vi "CREATE USER.vi"() -> ()   [LabVIEW 2021]
panel:
  in  "Cancel Button":bool
  in  "OK Button":bool
  in  "CONFIRM PASSWORD":string
  in  "PASSWORD":string
  in  "USER NAME":string
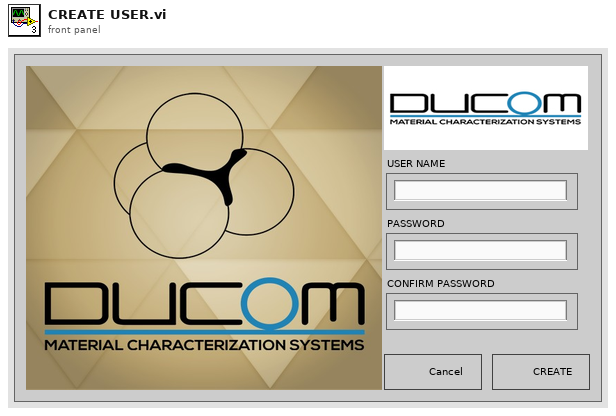
[diagram p1: front panel]
types:
  T1 = enum8{"Enabled", "Disabled", "Disabled and Grayed Out"}
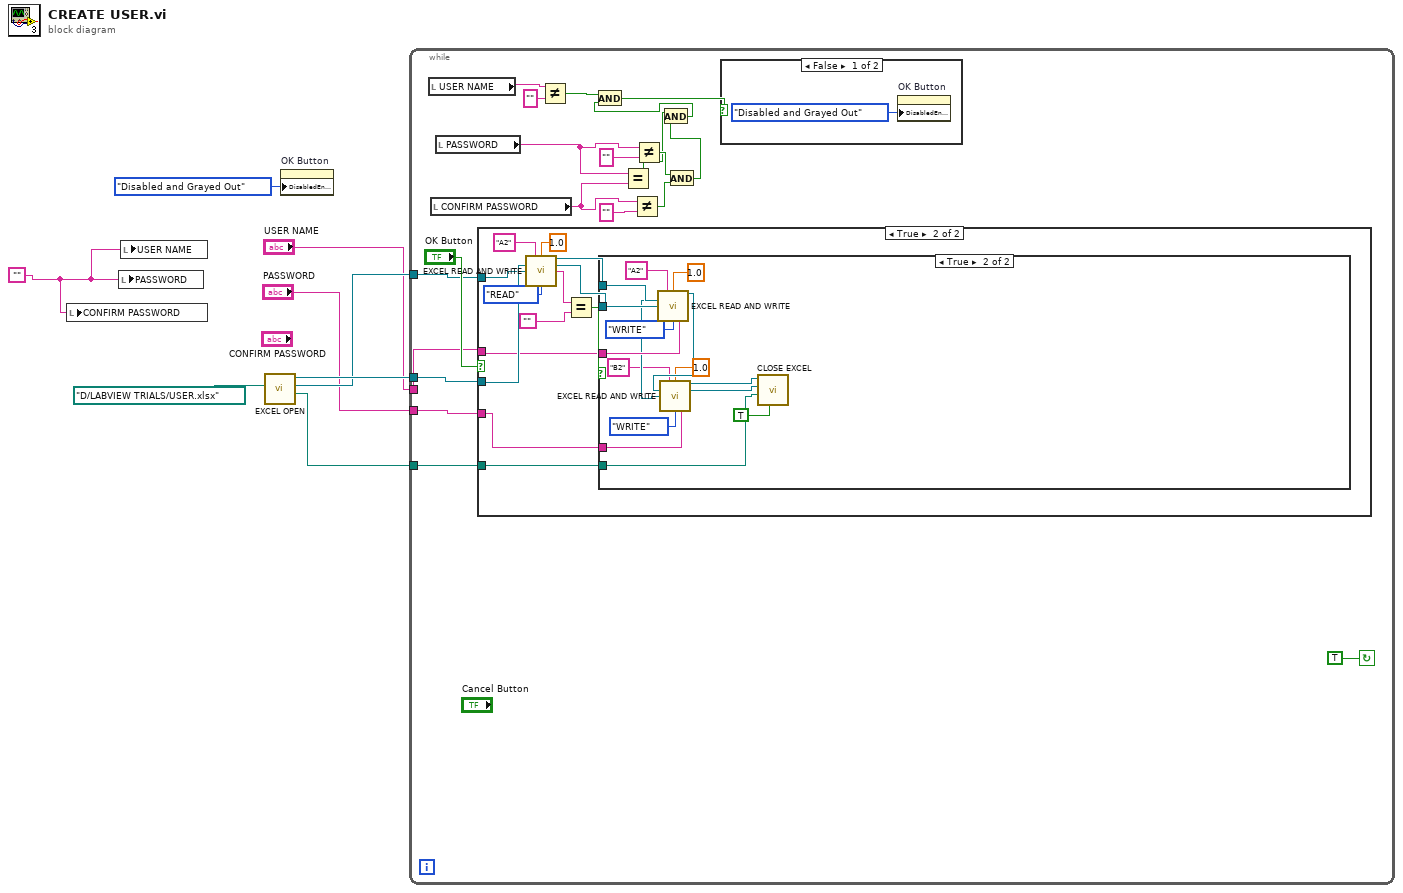
[diagram p0: block diagram]
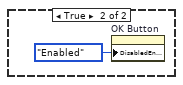
[diagram p4: hidden frame]
diagram:
  w7 = ""
  n1 = local write "CONFIRM PASSWORD"(w7) -> ()
  n2 = local write "PASSWORD"(w7) -> ()
  n3 = local write "USER NAME"(w7) -> ()
  n4 = call "EXCEL OPEN.vi"("PATH IN"=path "D:/LABVIEW TRIALS/USER.xlsx") -> ("PATH OUT"=w1:path, "WORKBOOK OUT"=w4:refnum<k7>, "Excel Application ref  out"=w5:refnum<k7>)  [unwired: 6 in, 2 out]
  n5 = property on="OK Button" class="Bool"("DisabledEnum"=T1."Disabled and Grayed Out" ("Disabled")) -> ()  [unwired: 2 in, 2 out]
  n6 = while {
    tunnel: w5 -> [w13]
    tunnel: w4 -> [w12]
    tunnel: "USER NAME" -> [w11]
    tunnel: "PASSWORD" -> [w10]
    tunnel: w1 -> [w9]
    stop <- TRUE continue-if-true
    n7 = local read "USER NAME"() -> (w17:string)
    n8 = local read "CONFIRM PASSWORD"() -> (w15:string)
    n9 = local read "PASSWORD"() -> (w16:string)
    n10 = case shown="True" "OK Button" {
      tunnel: w13 -> [_ w41]
      tunnel: w12 -> [_ w40]
      tunnel: w11 -> [_ w31]
      tunnel: w10 -> [_ w30]
      tunnel: w9 -> [_ w29]
      frame False {
      }
      frame True {
        n11 = call "EXCEL READ AND WRITE.vi"("CELL"="A2", "SHEET INDEX"=1.0, "Excel.Application REF in"=w41, "Excel._Workbook"=w40, "OPERATION"=enum16{"READ", "WRITE"}."READ") -> ("Excel Application ref out"=w33:refnum<k7>, "WORKBOOK REF OUT"=w32:refnum<k7>, "READING FROM EXCEL"=w36:string)  [unwired: 8 in]
        n12 = Equal?(x=w36, y="") -> (x = y?=w34:bool)
        n13 = case shown="True" w34 {
          tunnel: w33 -> [_ w57]
          tunnel: w32 -> [_ w56]
          tunnel: w31 -> [_ w52]
          tunnel: w30 -> [_ w46]
          tunnel: w29 -> [_ w43]
          frame False {
          }
          frame True {
            n14 = call "EXCEL READ AND WRITE.vi"("CELL"="A2", "SHEET INDEX"=1.0, "Excel.Application REF in"=w57, "Excel._Workbook"=w56, "OPERATION"=enum16{"READ", "WRITE"}."WRITE", "STRING TO WRITE"=w52) -> ("Excel Application ref out"=w51:refnum<k7>, "WORKBOOK REF OUT"=w50:refnum<k7>)  [unwired: 7 in, 1 out]
            n15 = call "EXCEL READ AND WRITE.vi"("CELL"="B2", "SHEET INDEX"=1.0, "Excel.Application REF in"=w51, "Excel._Workbook"=w50, "OPERATION"=enum16{"READ", "WRITE"}."WRITE", "STRING TO WRITE"=w46) -> ("Excel Application ref out"=w45:refnum<k7>, "WORKBOOK REF OUT"=w44:refnum<k7>)  [unwired: 7 in, 1 out]
            n16 = call "CLOSE EXCEL.vi"("SAVE"=TRUE, "File Path"=w43, "WORKBOOK REF IN"=w44, "APPLICATION REF IN"=w45) -> ()  [unwired: 8 in]
          }
        }
      }
    }
    n17 = Not Equal?(x=w17, y="") -> (x != y?=w21:bool)
    n18 = Equal?(x=w16, y=w15) -> (x = y?=w22:bool)
    n19 = Not Equal?(x=w15, y="") -> (x != y?=w24:bool)
    n20 = Not Equal?(x=w16, y="") -> (x != y?=w25:bool)
    n21 = And(x=w25, y=w24) -> (x .and. y?=w23:bool)
    n22 = And(x=w22, y=w23) -> (x .and. y?=w20:bool)
    n23 = And(x=w21, y=w20) -> (x .and. y?=w19:bool)
    n24 = case shown="False" w19 {
      frame False {
        n25 = property on="OK Button" class="Bool"("DisabledEnum"=T1."Disabled and Grayed Out" ("Disabled")) -> ()  [unwired: 2 in, 2 out]
      }
      frame True {
        n26 = property on="OK Button" class="Bool"("DisabledEnum"=T1."Enabled" ("Disabled")) -> ()  [unwired: 2 in, 2 out]
      }
    }
  }
